vi "AuMT8852B Instrument Status Query.vi"(8 "error in (no error)":errorcluster, 11 "VISA session":refnum<visa-resource-name>) -> (0 "error out":errorcluster, 2 "error code":i32, 3 "VISA session out":refnum<visa-resource-name>, 4 "Status":T1)   [LabVIEW 2017]
doc: "Anritsu MT8852B Bluetooth Tester\n\nReturns various information about the instrument's current state.\n\nOUTPUTS\nStatus:\nOperation mode - whether the instrument is in script, single test, signal generator. or CW Measurement mode\nSingle remote mode? - whether or not the insrument is in the single remote test state.\nSelected script - which script number is currently selected.\nSelected test - which test is selected in the current script.\nConnection? - whether or not a Bluetooth connection exists.\nReceiver gain range - selected gain range of the receiver.\n10MHz Reference Source - internal or external\nEUT TX Power - Min, Max, or intermediate\nSCO Channel <n> connected? - status of each SCO channel."
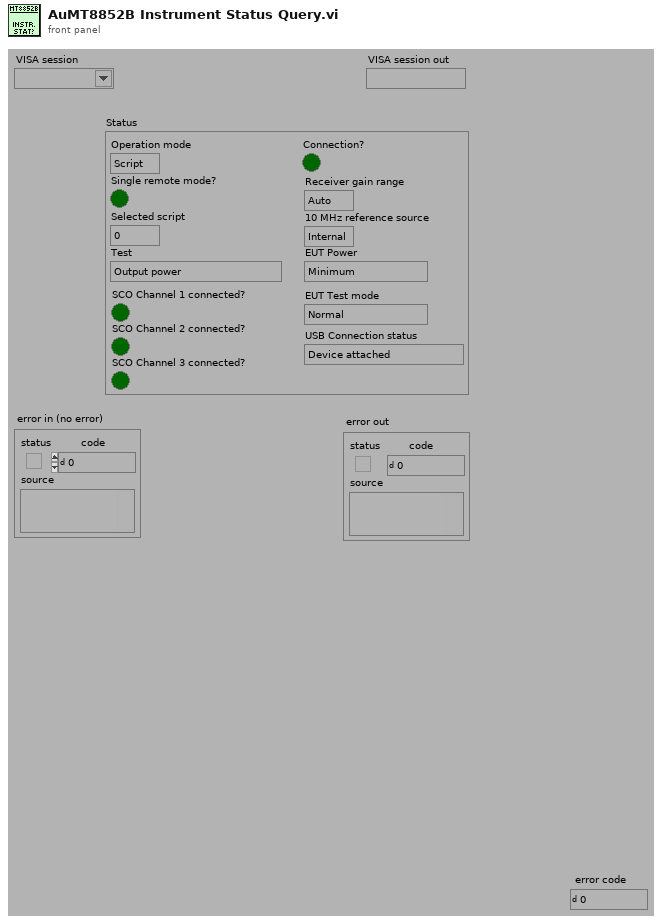
[diagram p1: front panel]
types:
  T1 = cluster{"Operation mode":enum16{"Script", "Single test", "Signal generator", "CW Measurement", "AFH Measurement", "EDR Signal generator", "EDR CW Measurement"}, "Single remote mode?":bool, "Selected script":i32, "Test":enum16{"Output power", "Power control", "Modulation characteristics", "Initial carrier", "Carrier drift", "Single slot sensitivity", "Multiple slot sensitivity", "Maximum input power", "Extended EDR tests", "EDR Relative transmit power", "EDR Carrier frequency stability", "EDR Differential phase encoding", "EDR Sensitivity", "EDR Floor sensitivity", "EDR Maximum input power"}, "Connection?":bool, "Receiver gain range":enum16{"Auto", "1", "2", "3", "4", "5", "6"}, "10 MHz reference source":enum16{"Internal", "External"}, "EUT Power":enum16{"Minimum", "Mid or unknown", "Maximum"}, "SCO Channel 1 connected?":bool, "SCO Channel 2 connected?":bool, "SCO Channel 3 connected?":bool, "EUT Test mode":enum16{"Normal", "Test"}, "USB Connection status":enum16{"Device attached", "Device removed", "Non Bluetooth device attached"}}
  T2 = enum16{"Simulate", "Range check", "Cache", "Query instrument status"}
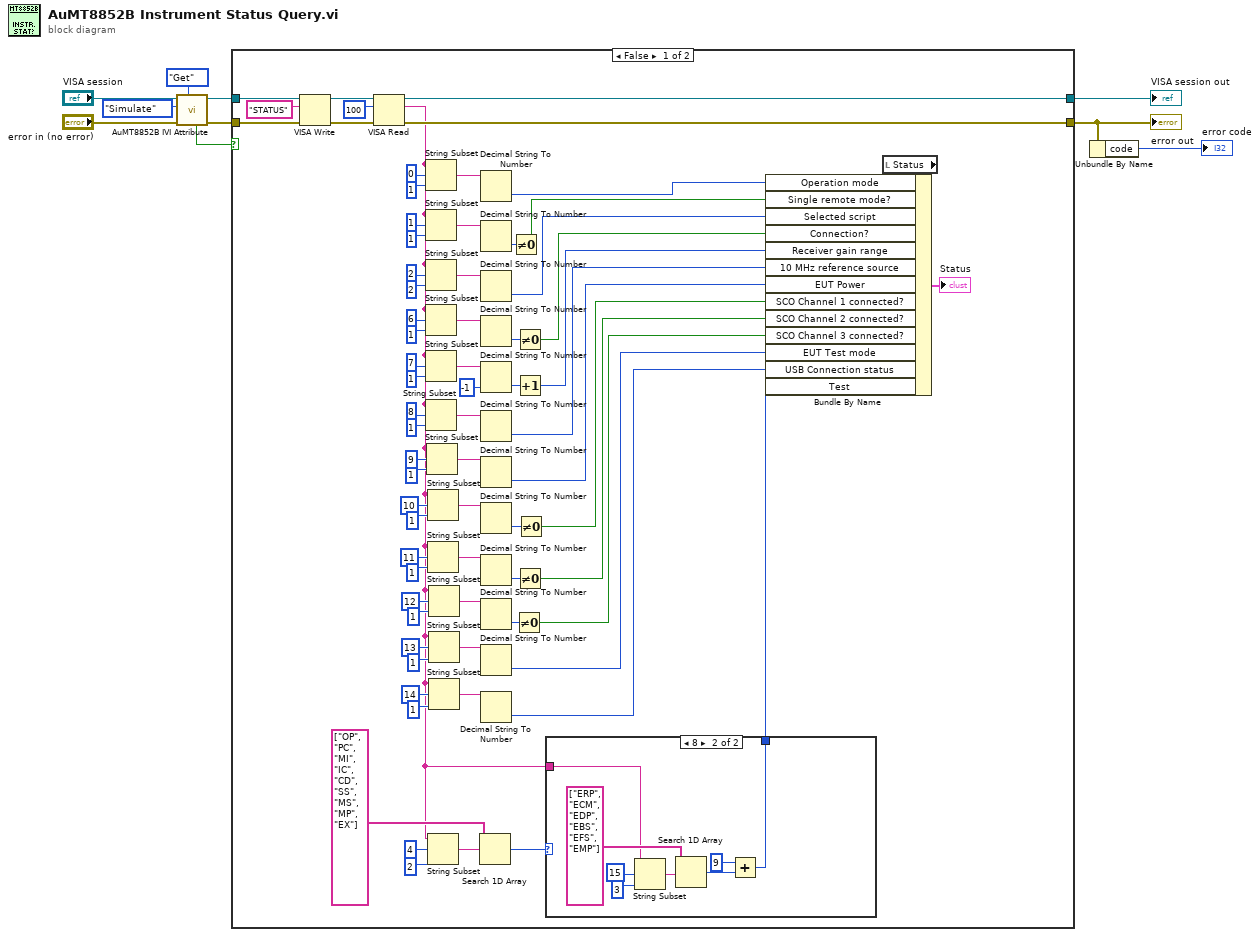
[diagram p0: block diagram]
diagram:
  n1 = call <instrlib>:"AuMT8852B IVI Attribute.vi"("Set/Get (Set)"=enum16{"Set", "Get"}."Get", "error in (no error)"="error in (no error)", "Flag (Simulate)"=T2."Simulate", "VISA session"="VISA session") -> ("error out"=w8:errorcluster, "VISA session out"=w9:refnum<visa-resource-name>, "Value out"=w3:bool)  [unwired: 5 in]
  n2 = case shown="False" w3 {
    tunnel: w9 -> [w82 w93]
    tunnel: w8 -> [w81 w92]
    tunnel: [w76 w93] -> w10
    tunnel: [w75 w92] -> w1
    frame False {
      n3 = VISA Write(VISA resource name=w82, write buffer="STATUS" ("write buffer (\"\")"), error in (no error)=w81) -> (VISA resource name out=w79:refnum<visa-resource-name>, error out=w78:errorcluster)  [unwired: 1 out]
      n4 = VISA Read(VISA resource name=w79, byte count=u32 100 ("byte count (0)"), error in (no error)=w78) -> (VISA resource name out=w76:refnum<visa-resource-name>, read buffer=w11:string, error out=w75:errorcluster)  [unwired: 1 out]
      n5 = String Subset(string=w11, offset (0)=0, length (rest)=1 ("length (rest)")) -> (substring=w72:string)
      n6 = String Subset(string=w11, offset (0)=1, length (rest)=1 ("length (rest)")) -> (substring=w62:string)
      n7 = String Subset(string=w11, offset (0)=2, length (rest)=2 ("length (rest)")) -> (substring=w61:string)
      n8 = String Subset(string=w11, offset (0)=6, length (rest)=1 ("length (rest)")) -> (substring=w60:string)
      n9 = String Subset(string=w11, offset (0)=7, length (rest)=1 ("length (rest)")) -> (substring=w59:string)
      n10 = String Subset(string=w11, offset (0)=8, length (rest)=1 ("length (rest)")) -> (substring=w52:string)
      n11 = String Subset(string=w11, offset (0)=9, length (rest)=1 ("length (rest)")) -> (substring=w49:string)
      n12 = String Subset(string=w11, offset (0)=10, length (rest)=1 ("length (rest)")) -> (substring=w42:string)
      n13 = String Subset(string=w11, offset (0)=11, length (rest)=1 ("length (rest)")) -> (substring=w41:string)
      n14 = String Subset(string=w11, offset (0)=4, length (rest)=2 ("length (rest)")) -> (substring=w14:string)
      n15 = String Subset(string=w11, offset (0)=12, length (rest)=1 ("length (rest)")) -> (substring=w36:string)
      n16 = String Subset(string=w11, offset (0)=13, length (rest)=1 ("length (rest)")) -> (substring=w31:string)
      n17 = String Subset(string=w11, offset (0)=14, length (rest)=1 ("length (rest)")) -> (substring=w20:string)
      n18 = Search 1D Array(1D array=string[] ["OP", "PC", "MI", "IC", "CD", "SS", "MS", "MP", "EX"] ("Array Constant"), element=w14) -> (index of element=w13:i32)  [unwired: 1 in]
      n19 = Decimal String To Number(string=w72) -> (number=w63:i32)  [unwired: 2 in, 1 out]
      n20 = Decimal String To Number(string=w62) -> (number=w58:i32)  [unwired: 2 in, 1 out]
      n21 = Decimal String To Number(string=w61) -> (number=w56:i32)  [unwired: 2 in, 1 out]
      n22 = Decimal String To Number(string=w60) -> (number=w55:i32)  [unwired: 2 in, 1 out]
      n23 = Decimal String To Number(string=w59, default (0L)=-1) -> (number=w53:i32)  [unwired: 1 in, 1 out]
      n24 = Decimal String To Number(string=w52) -> (number=w27:i32)  [unwired: 2 in, 1 out]
      n25 = Decimal String To Number(string=w49) -> (number=w26:i32)  [unwired: 2 in, 1 out]
      n26 = Decimal String To Number(string=w42) -> (number=w35:i32)  [unwired: 2 in, 1 out]
      n27 = Decimal String To Number(string=w41) -> (number=w34:i32)  [unwired: 2 in, 1 out]
      n28 = Decimal String To Number(string=w36) -> (number=w33:i32)  [unwired: 2 in, 1 out]
      n29 = Decimal String To Number(string=w31) -> (number=w22:i32)  [unwired: 2 in, 1 out]
      n30 = Decimal String To Number(string=w20) -> (number=w18:i32)  [unwired: 2 in, 1 out]
      n31 = Not Equal To 0?(x=w58) -> (x != 0?=w57:bool)
      n32 = Not Equal To 0?(x=w33) -> (x != 0?=w23:bool)
      n33 = Not Equal To 0?(x=w55) -> (x != 0?=w29:bool)
      n34 = Increment(x=w53) -> (x+1=w28:i32)
      n35 = Not Equal To 0?(x=w34) -> (x != 0?=w24:bool)
      n36 = Not Equal To 0?(x=w35) -> (x != 0?=w25:bool)
      n37 = case shown="8" w13 {
        selector: w13 -> [w83 _]
        tunnel: [w83 w84] -> w12
        tunnel: w11 -> [_ w87]
        frame 0..7, Default {
        }
        frame 8 {
          n38 = String Subset(string=w87, offset (0)=15, length (rest)=3 ("length (rest)")) -> (substring=w90:string)
          n39 = Search 1D Array(1D array=string[] ["ERP", "ECM", "EDP", "EBS", "EFS", "EMP"] ("Array Constant"), element=w90) -> (index of element=w86:i32)  [unwired: 1 in]
          n40 = Add(x=9, y=w86) -> (x+y=w84:i32)
        }
      }
      n41 = local read "Status"() -> (w45:T1)
      n42 = Bundle By Name(cluster=w45, "Operation mode"=w63, "Single remote mode?"=w57, "Selected script"=w56, "Connection?"=w29, "Receiver gain range"=w28, "10 MHz reference source"=w27, "EUT Power"=w26, "SCO Channel 1 connected?"=w25, "SCO Channel 2 connected?"=w24, "SCO Channel 3 connected?"=w23, "EUT Test mode"=w22, "USB Connection status"=w18, "Test"=w12) -> (→"Status":T1)
    }
    frame True {
    }
  }
  "error out" <- w1
  "VISA session out" <- w10
  n43 = Unbundle By Name(w1) -> ("code"=→"error code":i32)
